vi "Set Rig.vi"(8 "error in (no error)":errorcluster, 9 "Rig":string, 11 "Tosca in":refnum<class "Parameters.lvclass">) -> (0 "error out":errorcluster, 3 "Tosca out":refnum<class "Parameters.lvclass">)   [LabVIEW 2015, in "Parameters.lvclass"]
uses:
  Parameters.lvclass
  Parameters.lvclass/Parameters.ctl
  State/State.lvclass
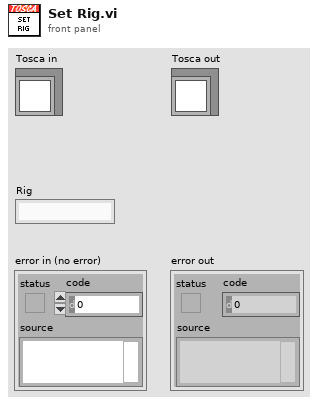
[diagram p1: front panel]
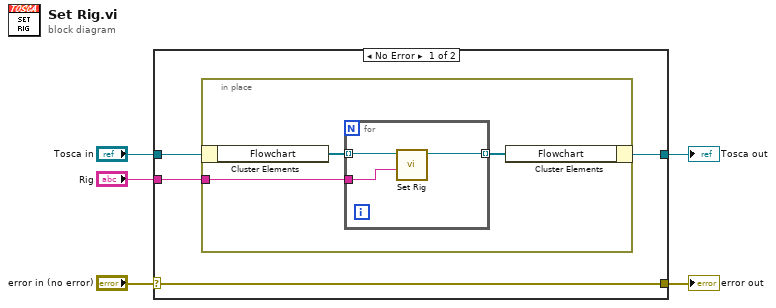
[diagram p0: block diagram]
diagram:
  n1 = case shown="No Error" "error in (no error)" {
    selector: "error in (no error)" -> [w9 w17]
    tunnel: [w9 w17] -> w4
    tunnel: [w7 w16] -> w2
    tunnel: "Tosca in" -> [w8 w16]
    tunnel: "Rig" -> [w6 _]
    frame No Error {
      n2 = in-place {
        in-place-border: w6 -> [w10]
        n3 = in-place-cluster #1(w8) -> ("Flowchart"=w12:refnum<class "State.lvclass">[])
        n4 = for {
          tunnel: w12 -> [w15] mode=indexing
          tunnel: [w14] -> w11 mode=indexing
          tunnel: w10 -> [w13]
          n5 = call "Set Rig.vi"("Rig"=w13, "State in"=w15) -> ("State out"=w14:refnum<class "State.lvclass">)  [unwired: 8 in, 1 out]
        }
        n6 = in-place-cluster #1("Flowchart"=w11) -> (w7:refnum<class "Parameters.lvclass">)
      }
    }
    frame Error {
    }
  }
  "error out" <- w4
  "Tosca out" <- w2
